vi "command error.vi"(4 "Error Details":string, 5 "Comment":string, 7 "5 Sec Countdown":bool) -> ()   [LabVIEW 2020]
doc: "[Ver 1.00]\n\nDESCRIPTION\nReuseable Component. This vi detects where a command error occured and displays a warning message. Use the Call Chain to work out where the error occured.\n__________________________________\nVERSION CONTROL\nV1.00 New Version SSDC 19/01/2000"
panel:
  out "Time":string
  in  "OK":bool
  out "Call Chain":string[](array[string])
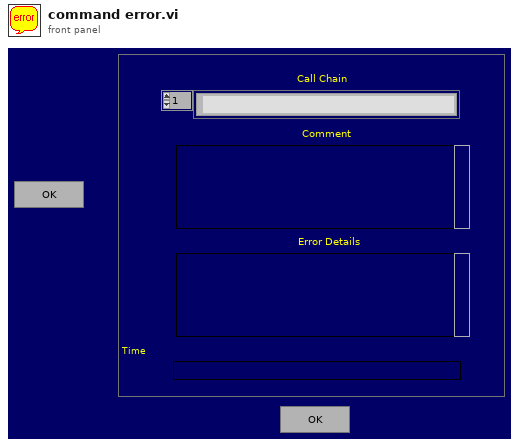
[diagram p1: front panel]
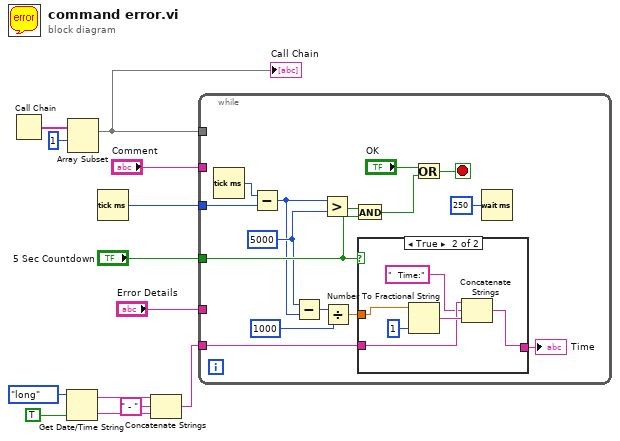
[diagram p0: block diagram]
diagram:
  n1 = Call Chain() -> (call chain=w13:string[])
  n2 = Get Date/Time String(date format (0)=enum16{"short", "long", "abbreviated"}."long", want seconds? (F)=TRUE) -> (date string=w8:string, time string=w7:string)  [unwired: 1 in]
  n3 = Array Subset(array=w13, index=1 ("Array Index")) -> (w12:string[])  [unwired: 1 in]
  "Call Chain" <- w12
  n4 = Tick Count (ms)() -> (millisecond timer value=w3:u32)
  n5 = Concatenate Strings(w8, " - " ("string"), w7) -> (w5:string)
  n6 = while {
    tunnel: w12 -> [_]
    tunnel: w5 -> [w20]
    tunnel: "Comment" -> [_]
    tunnel: w3 -> [w26]
    tunnel: "5 Sec Countdown" -> [w21]
    tunnel: "Error Details" -> [_]
    stop <- w25 stop-if-true
    w19 = u32 5000 ("y")
    n7 = Tick Count (ms)() -> (millisecond timer value=w27:u32)
    n8 = Subtract(x=w27, y=w26) -> (x-y=w18:u32)
    n9 = Subtract(x=w19, y=w18) -> (x-y=w16:u32)
    n10 = Greater?(x=w18, y=w19) -> (0:w23:bool)
    n11 = Divide(x=w16, y=u32 1000) -> (x/y=w14:dbl)
    n12 = And(x=w23, y=w21) -> (x .and. y?=w22:bool)
    n13 = case shown="True" w21 {
      tunnel: w20 -> [w29 w34]
      tunnel: [w29 w32] -> w17
      tunnel: w14 -> [_ w31]
      frame False {
      }
      frame True {
        n14 = Number To Fractional String(number=w31, precision (6)=i16 1) -> (F-format string=w35:string)  [unwired: 2 in]
        n15 = Concatenate Strings(w34, "  Time:" ("string"), w35) -> (w32:string)
      }
    }
    "Time" <- w17
    n16 = Or(x="OK", y=w22) -> (x .or. y?=w25:bool)
    n17 = Wait (ms)(milliseconds to wait=u32 250) -> ()  [unwired: 1 out]
  }
